vi "Obtain Status.vi"(8 "Error In":errorcluster, 11 "Configuration In":refnum<class "Configuration.lvclass">) -> (0 "Error Out":errorcluster, 1 "Status":string, 2 "Page":T1(ring), 3 "Configuration out":refnum<class "Configuration.lvclass">)   [LabVIEW 2019, in "Configuration.lvclass"]
doc: "The VI decides the page to be set and the current status."
uses:
  Configuration.lvclass
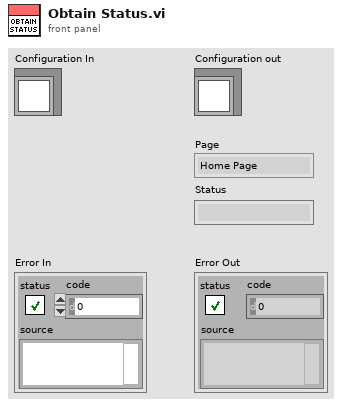
[diagram p1: front panel]
types:
  T1 = enum32{"Home Page", "Mode Page", "Configuration Page", "Input Page", "Result Page"}
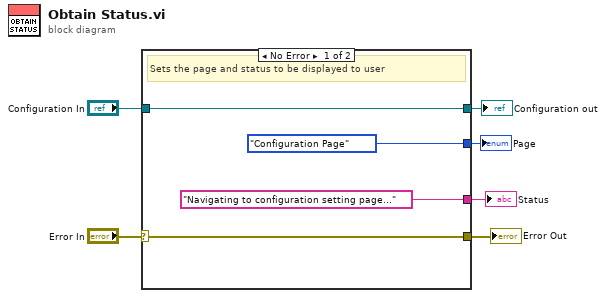
[diagram p0: block diagram]
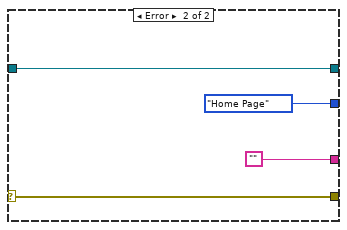
[diagram p2: hidden frame]
diagram:
  n1 = case shown="No Error" "Error In" {
    selector: "Error In" -> [w9 w14]
    tunnel: [w9 w14] -> w5
    tunnel: [w10 w13] -> w3
    tunnel: "Configuration In" -> [w10 w13]
    tunnel: [T1."Configuration Page" ("Page") T1."Home Page" ("Page")] -> w2
    tunnel: ["Navigating to configuration setting page..." ""] -> w1
    frame No Error {
      # "Sets the page and status to be displayed to user"
    }
    frame Error {
    }
  }
  "Error Out" <- w5
  "Configuration out" <- w3
  "Page" <- w2
  "Status" <- w1
